vi "配置读取.vi"(8 "error in (no error)":errorcluster caption="错误输入（无错误）", 11 "TimingControl 输入":refnum<class "TimingControl.lvclass">) -> (0 "error out":errorcluster caption="错误输出", 3 "TimingControl 输出":refnum<class "TimingControl.lvclass">)   [LabVIEW 2016, in "TimingControl.lvclass"]
uses:
  TimingControl.lvclass
  TimingControl.lvclass/TimingControl.ctl
  <vilib>/Utility/xml.llb/Read From XML File(string).vi
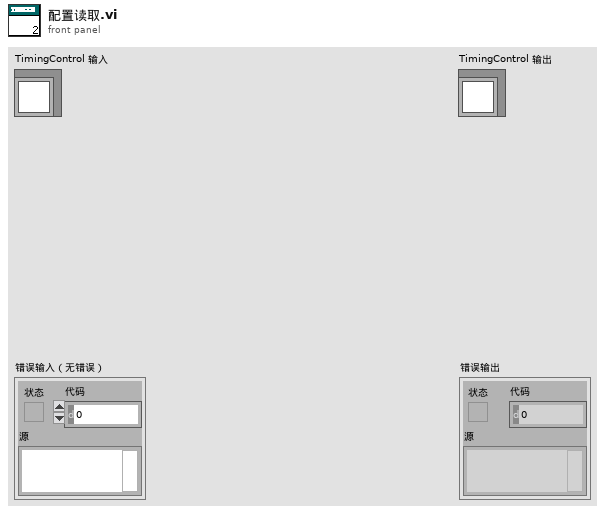
[diagram p1: front panel]
types:
  T1 = typedef "TimingControl.lvclass/State Data.ctl" = cluster{"仪器时间":timestamp, "仪器运行状态":bool, "配置文件路径":path, "测量参数":u16, "测试状态":cluster{"启动时间":timestamp, "结束时间":timestamp, "启动次数":dbl}, "配置信息":cluster{"每周启动":T2, "每月启动":T3, "周期模式":T4, "测量参数":T5, "定点周期":T6, "间隔启动":T8}}
  T2 = typedef "TimingControl.lvclass/每周启动.ctl" = enum16{"关闭", "周日", "周一", "周二", "周三", "周四", "周五", "周六"}
  T3 = typedef "TimingControl.lvclass/每月启动.ctl" = enum16{"关闭", "1号", "2号", "3号", "4号", "5号", "6号", "7号", "8号", "9号", "10号", "11号", "12号", "13号", "14号", "15号", "16号", "17号", "18号", "19号", "20号", "21号", "22号", "23号", "24号", "25号", "26号", "27号", "28号", "29号", "30号", "31号"}
  T4 = typedef "TimingControl.lvclass/周期模式设置.ctl" = enum16{"不启用", "定点模式", "间隔模式"}
  T5 = typedef "TimingControl.lvclass/测量参数.ctl" = u16
  T6 = typedef "TimingControl.lvclass/定点周期设置.ctl" = cluster{"启动命令":T7, "启动命令 2":T7, "启动命令 3":T7, "启动命令 4":T7, "启动命令 5":T7, "启动命令 6":T7, "启动命令 7":T7, "启动命令 8":T7, "启动命令 9":T7, "启动命令 10":T7, "启动命令 11":T7, "启动命令 12":T7, "启动命令 13":T7, "启动命令 14":T7, "启动命令 15":T7, "启动命令 16":T7, "启动命令 17":T7, "启动命令 18":T7, "启动命令 19":T7, "启动命令 20":T7, "启动命令 21":T7, "启动命令 22":T7, "启动命令 23":T7, "启动命令 24":T7}
  T7 = typedef "TimingControl.lvclass/启动命令选择.ctl" = enum16{"", "水样测试", "标样核查", "零点核查", "跨度核查", "空白测试", "平行样测试", "加标回收", "空白校准", "标样校准", "初始化(清洗)"}
  T8 = typedef "TimingControl.lvclass/间隔启动设置.ctl" = cluster{"启动命令":T7, "启动间隔":dbl, "启动次数":i32}
  T9 = cluster{"每周启动":T2, "每月启动":T3, "周期模式":T4, "测量参数":T5, "定点周期":T6, "间隔启动":T8}
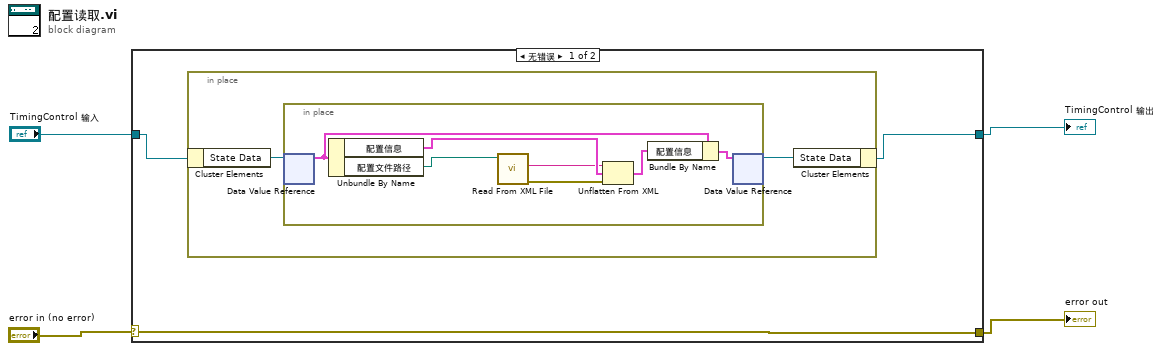
[diagram p0: block diagram]
diagram:
  n1 = case shown="无错误" "error in (no error)" {
    selector: "error in (no error)" -> [w7 w18]
    tunnel: [w7 w18] -> w3
    tunnel: [w5 w17] -> w1
    tunnel: "TimingControl 输入" -> [w6 w17]
    frame No Error {
      n2 = in-place {
        n3 = in-place-cluster #1(w6) -> ("State Data"=w9:refnum<data-value>)
        n4 = in-place {
          n5 = in-place-dvr #2(w9) -> (w15:T1)  [unwired: 1 out]
          n6 = Unbundle By Name(w15) -> ("配置信息"=w14:T9, "配置文件路径"=w12:path)
          n7 = call-poly <vilib>:"Read From XML File.vi"("XML File Path"=w12) -> ("error out"=w10:errorcluster, "XML Elements"=w11:string)  [unwired: 8 in, 1 out]
          n8 = Unflatten From XML(xml string=w11, type=w14, error in (no error)=w10) -> (value=w13:T9)  [unwired: 1 out]
          n9 = Bundle By Name(cluster=w15, "配置信息"=w13) -> (w16:T1)
          n10 = in-place-dvr #2(w16) -> (w8:refnum<data-value>)  [unwired: 1 out]
        }
        n11 = in-place-cluster #1("State Data"=w8) -> (w5:refnum<class "TimingControl.lvclass">)
      }
    }
    frame Error {
    }
  }
  "error out" <- w3
  "TimingControl 输出" <- w1
